vi "labviewArduino_1.vi"() -> ()   [LabVIEW 2017]
uses:
  <vilib>/MakerHub/LINX/Public/Peripherals/Digital/Digital Write N Chans.vi
  <vilib>/MakerHub/LINX/Private/Local IO/LinxDigitalWrite.vi
  <vilib>/MakerHub/LINX/Public/Utilities/Check Channel.vi
  <vilib>/MakerHub/LINX/Public/Utilities/Open Serial.vi
  <vilib>/MakerHub/LINX/Private/Utilties/Generate Error.vi
  <vilib>/Utility/file.llb/Write To Spreadsheet File (DBL).vi
  <vilib>/MakerHub/LINX/LMH-LINX.lvlib
panel:
  out "error out":errorcluster
  out "Result (V - I)":dbl[][](array[numeric]) format="%^#.6e"
  out "XY Graph 3":cluster{dbl[], dbl[]}(graph)
  in  "SweepSettings":T1 {"Vstep (V)" format="%.3f"; "Vstop (V)" format="%.3f"; "Vstart (V)" format="%.3f"}
  in  "Amount of modules connected":enum16{"1", "2", "3", "4", "5", "6"}(ring)
  in  "Start Button":bool
  in  "Time between measurements(s)":u32
  in  "Stop Button 2":bool
  in  "Time High Voltage Source is active (s)":u32
  in  "High voltage Source polarity":enum16{"-0+", "0-+", "-+0", "+0-"}(ring)
  out "Loop Rate (Hz)":u32
  in  "Serial Port":refnum<visa-resource-name>
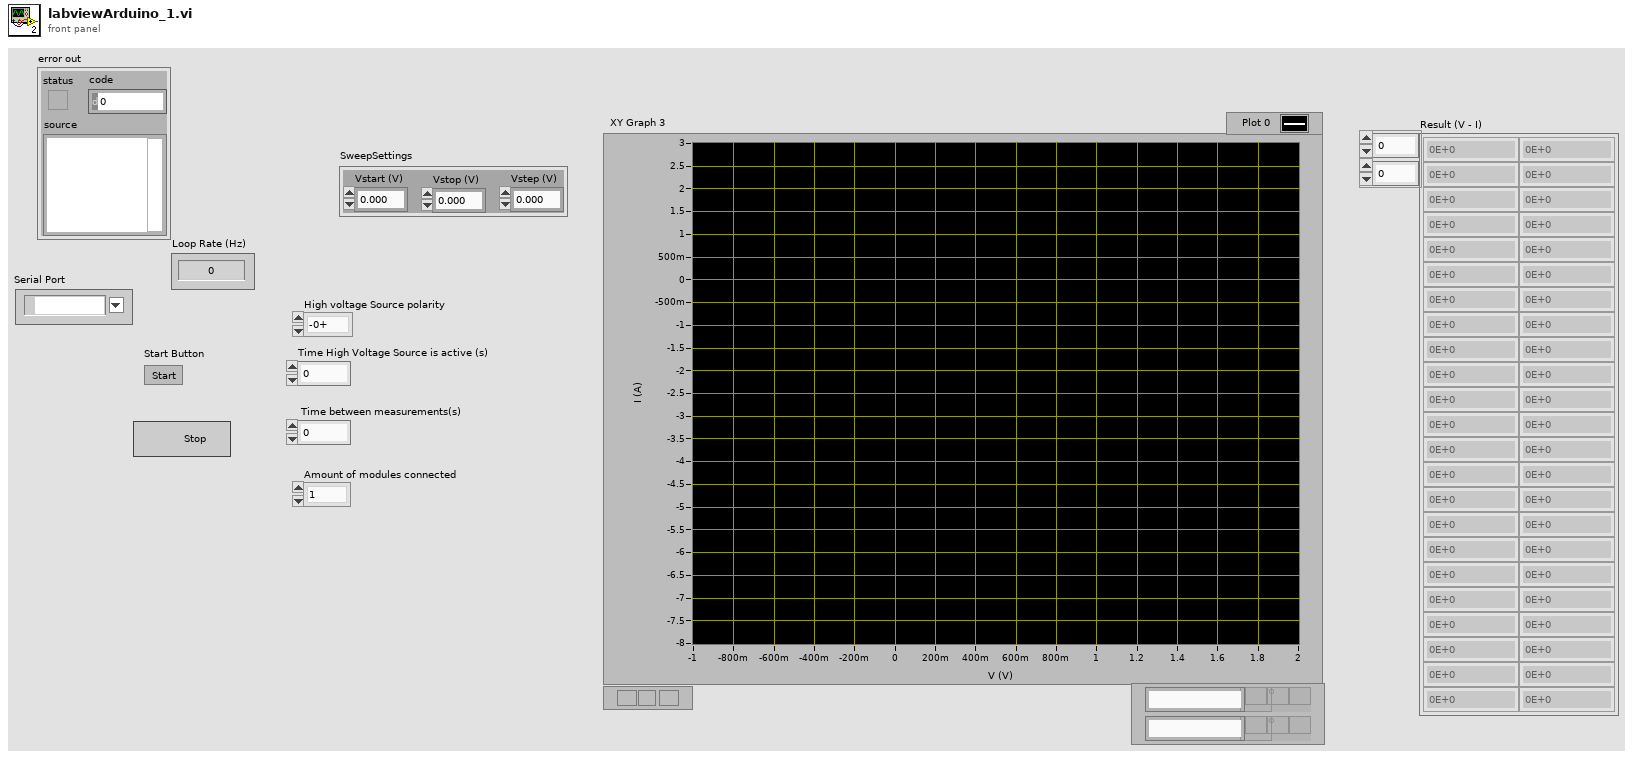
[diagram p1: front panel]
types:
  T1 = cluster{"Vstart (V)":dbl, "Vstop (V)":dbl, "Vstep (V)":dbl}
  T2 = enum16{"Rest", "HV Source On", "Measure", "Relay 1", "Relay 2", "Relay 3", "Relay 4", "Relay 5", "Relay 6"}
  T3 = enum16{"Rest", "HV Source On", "Relay 1", "Relay 2", "Relay 3", "Relay 4", "Relay 5", "Relay 6"}
  T4 = typedef "LMH-LINX.lvlib/LINX Ref.ctl" = cluster{"IO":T5, "Interface":T6, "LINX Device Config":T7}
  T5 = typedef "LMH-LINX.lvlib/Platform.ctl" = enum16{"Remote", "Local"}
  T6 = typedef "LMH-LINX.lvlib/Interface.ctl" = enum16{"Serial", "TCP"}
  T7 = typedef "LMH-LINX.lvlib/Device.lvlib/LINX Device Config.ctl" = cluster{"Interface":T6, "COM Port":refnum<visa-resource-name>, "TCP Configuration":T8, "Device Family":u8, "Device ID":u8, "Device Name":string, "TCP Ref":refnum<k5>, "Channels":T9}
  T8 = typedef "LMH-LINX.lvlib/Device.lvlib/TCP Config.ctl" = cluster{"IP Address":string, "Port":u16}
  T9 = typedef "LMH-LINX.lvlib/Channels.ctl" = cluster{"DI":u8[], "DO":u8[], "AI":u8[], "AO":u8[], "PWM":u8[], "QE":u8[], "UART":u8[], "I2C 2":u8[], "SPI":u8[], "CAN":u8[], "Servo":u8[], "AI Ref (V)":dbl, "AI Resolution (Bits)":u8, "AO Ref (V)":dbl, "AO Resolution (Bits)":u8}
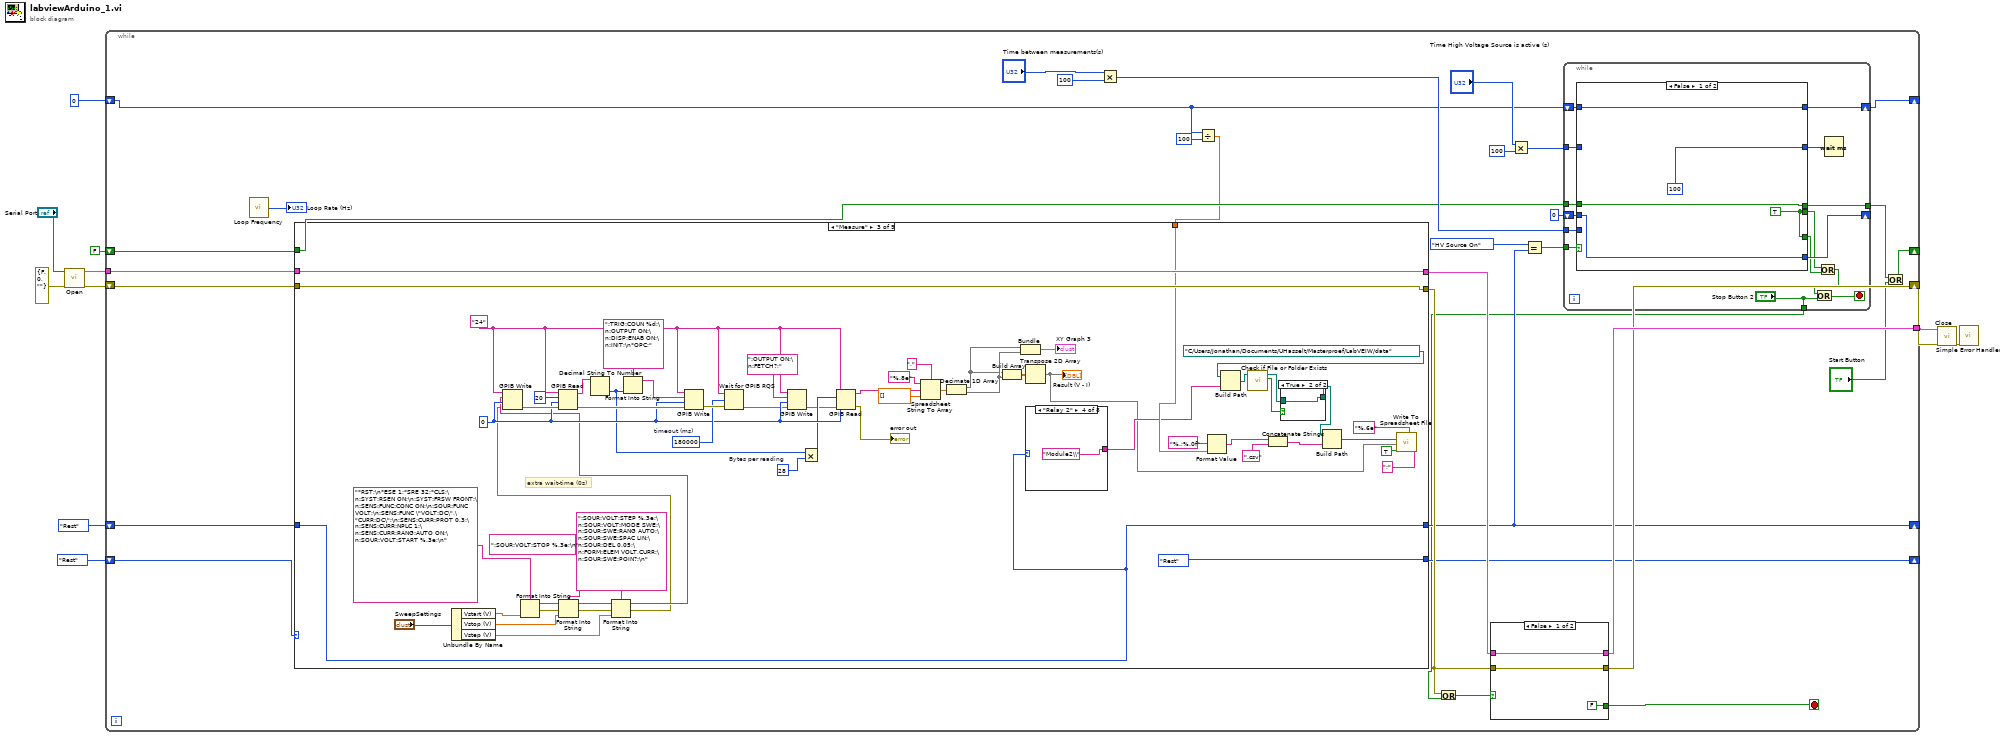
[diagram p0: block diagram]
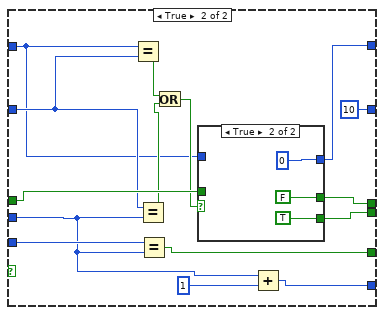
[diagram p2: hidden frame]
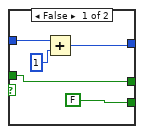
[diagram p3: hidden frame]
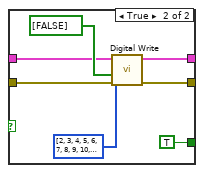
[diagram p4: hidden frame]
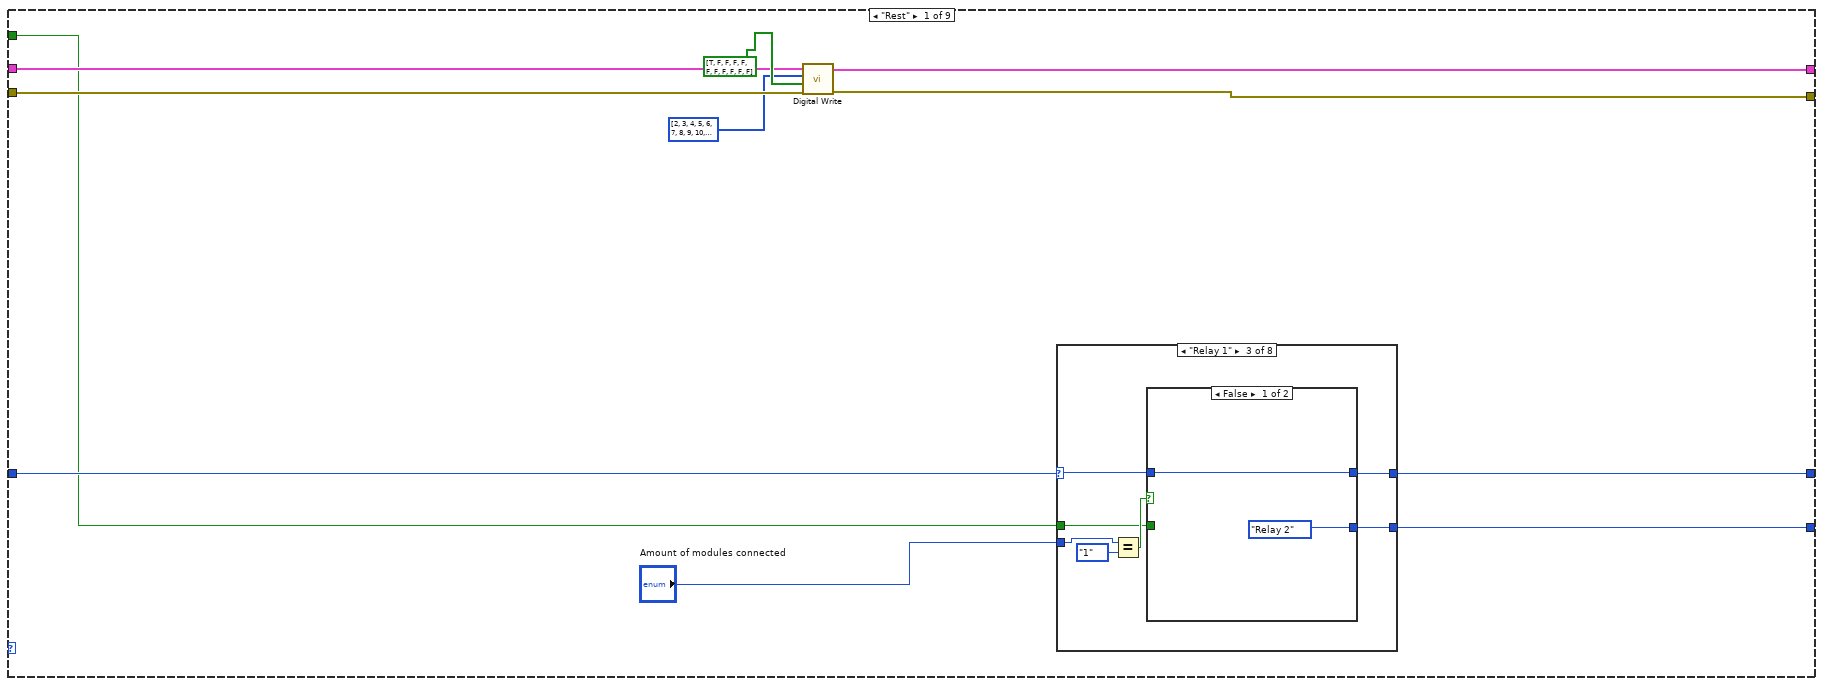
[diagram p5: hidden frame]
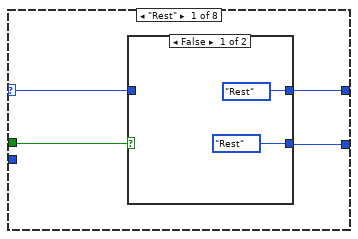
[diagram p6: hidden frame]
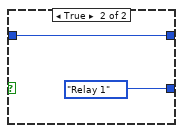
[diagram p7: hidden frame]
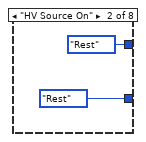
[diagram p8: hidden frame]
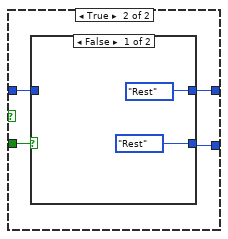
[diagram p9: hidden frame]
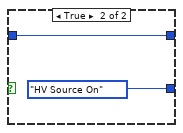
[diagram p10: hidden frame]
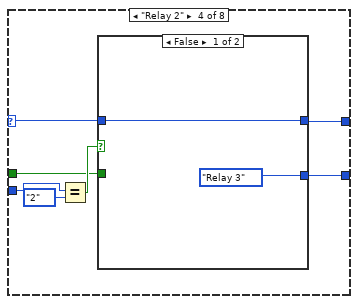
[diagram p11: hidden frame]
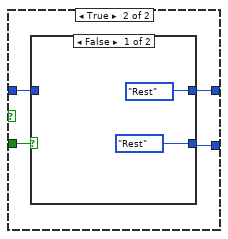
[diagram p12: hidden frame]
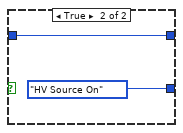
[diagram p13: hidden frame]
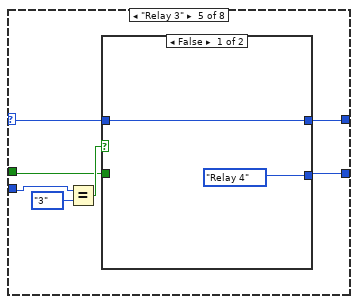
[diagram p14: hidden frame]
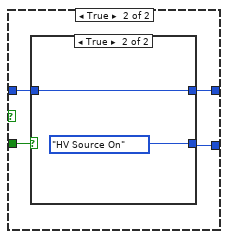
[diagram p15: hidden frame]
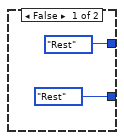
[diagram p16: hidden frame]
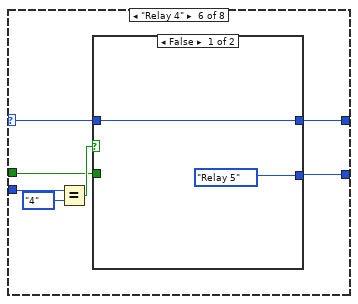
[diagram p17: hidden frame]
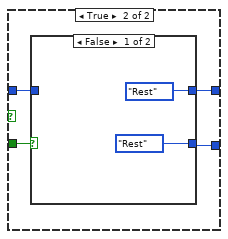
[diagram p18: hidden frame]
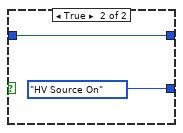
[diagram p19: hidden frame]
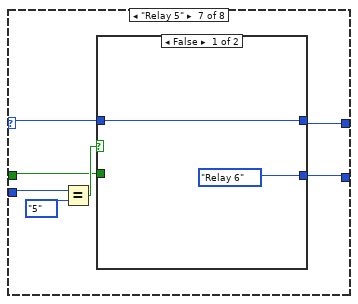
[diagram p20: hidden frame]
diagram:
  n1 = call-poly <vilib>:"Open.vi"("Error In"=errorcluster {"status"=FALSE, "code"=0, "source"=""}, "Serial Port"="Serial Port") -> ("Error Out"=w10:errorcluster, "LINX Resource"=w11:T4)  [unwired: 7 in, 1 out]
  n2 = while {
    tunnel: w11 -> [w41]
    tunnel: [w36] -> w9
    shift-right: [w35] -> w8
    shift-left: w10 -> [w40]
    shift-right: [w32] -> _
    shift-left: T2."Rest" ("Enum 2") -> [w17]
    shift-right: [w31] -> _
    shift-left: T3."Rest" ("Enum 2") -> [w33]
    shift-right: [w18] -> _
    shift-left: u32 0 ("y") -> [w14]
    shift-right: [w16] -> _
    shift-left: FALSE -> [w15]
    stop <- w27 stop-if-true
    n3 = call <vilib>:"Loop Frequency.vi"() -> ("Loop Rate (Hz)"=→"Loop Rate (Hz)":u32)
    n4 = Multiply(x="Time between measurements(s)", y=u32 100) -> (x*y=w21:u32)
    n5 = Divide(x=w14, y=u32 100) -> (x/y=w12:dbl)
    n6 = case shown="\"Measure\"" w17 {
      tunnel: [w106 T2."Rest" ("Enum 2") T2."Rest" ("Enum 2") T2."Measure" ("Enum 2") T2."Measure" ("Enum 2") T2."Measure" ("Enum 2") T2."Measure" ("Enum 2") T2."Measure" ("Enum 2") T2."Measure" ("Enum 2")] -> w32
      tunnel: w41 -> [w104 w231 w313 w331 w337 w347 w355 w363 w371]
      tunnel: w40 -> [w103 w230 w312 w330 w336 w346 w354 w362 w370]
      tunnel: [w102 w229 w312 w329 w338 w345 w352 w361 w369] -> w37
      tunnel: [w101 w226 w313 w328 w339 w344 w353 w360 w368] -> w38
      tunnel: [w99 T3."HV Source On" ("Enum 2") w311 T3."Relay 1" ("Enum 2") T3."Relay 2" ("Enum 2") T3."Relay 3" ("Enum 2") T3."Relay 4" ("Enum 2") T3."Relay 5" ("Enum 2") T3."Relay 6" ("Enum 2")] -> w31
      tunnel: w33 -> [w100 _ w311 _ _ _ _ _ _]
      tunnel: w15 -> [w98 _ _ _ _ _ _ _ _]
      tunnel: w12 -> [_ _ w306 _ _ _ _ _ _]
      frame "Rest" {
        n7 = call-poly <vilib>:"Digital Write.vi"("Error In"=w103, "Values"=bool[] [TRUE, FALSE, FALSE, FALSE, FALSE, FALSE, FALSE, FALSE, FALSE, FALSE, FALSE], "DO Channels"=u8[] [2, 3, 4, 5, 6, 7, 8, 9, 10, 11, 12, 13], "LINX Resource"=w104) -> ("Error Out"=w102:errorcluster, "LINX Resource"=w101:T4)  [unwired: 6 in]
        n8 = case shown="\"Relay 1\"" w100 {
          selector: w100 -> [w109 _ w119 w138 w155 w169 w187 w207]
          tunnel: [w108 T2."Rest" ("Enum 2") w118 w135 w152 w171 w189 w208] -> w106
          tunnel: [w110 T3."Rest" ("Enum 2") w117 w136 w153 w172 w188 w206] -> w99
          tunnel: w98 -> [w107 _ w120 w137 w154 w170 w186 w205]
          tunnel: "Amount of modules connected" -> [_ _ w121 w134 w151 w168 w185 w204]
          frame "Rest" {
            n9 = case shown="False" w107 {
              tunnel: [T2."Rest" ("Enum 2") T2."Relay 1" ("Enum 2")] -> w108
              tunnel: [T3."Rest" ("Enum 2") w113] -> w110
              tunnel: w109 -> [_ w113]
              frame False {
              }
              frame True {
              }
            }
          }
          frame "HV Source On" {
          }
          frame "Relay 1" {
            n10 = Equal?(x=w121, y=enum16{"1", "2", "3", "4", "5", "6"}."1") -> (x = y?=w122:bool)
            n11 = case shown="False" w122 {
              tunnel: [T2."Relay 2" ("Enum 2") w129] -> w118
              tunnel: w119 -> [w125 w128]
              tunnel: [w125 w127] -> w117
              tunnel: w120 -> [_ w126]
              frame False {
              }
              frame True {
                n12 = case shown="False" w126 {
                  tunnel: [T2."Rest" ("Enum 2") T2."HV Source On" ("Enum 2")] -> w129
                  tunnel: [T3."Rest" ("Enum 2") w133] -> w127
                  tunnel: w128 -> [_ w133]
                  frame False {
                  }
                  frame True {
                  }
                }
              }
            }
          }
          frame "Relay 2" {
            n13 = Equal?(x=w134, y=enum16{"1", "2", "3", "4", "5", "6"}."2") -> (x = y?=w139:bool)
            n14 = case shown="False" w139 {
              tunnel: [T2."Relay 3" ("Enum 2") w146] -> w135
              tunnel: w138 -> [w142 w145]
              tunnel: [w142 w144] -> w136
              tunnel: w137 -> [_ w143]
              frame False {
              }
              frame True {
                n15 = case shown="False" w143 {
                  tunnel: [T2."Rest" ("Enum 2") T2."HV Source On" ("Enum 2")] -> w146
                  tunnel: [T3."Rest" ("Enum 2") w150] -> w144
                  tunnel: w145 -> [_ w150]
                  frame False {
                  }
                  frame True {
                  }
                }
              }
            }
          }
          frame "Relay 3" {
            n16 = Equal?(x=w151, y=enum16{"1", "2", "3", "4", "5", "6"}."3") -> (x = y?=w156:bool)
            n17 = case shown="False" w156 {
              tunnel: [T2."Relay 4" ("Enum 2") w163] -> w152
              tunnel: w155 -> [w159 w162]
              tunnel: [w159 w161] -> w153
              tunnel: w154 -> [_ w160]
              frame False {
              }
              frame True {
                n18 = case shown="True" w160 {
                  tunnel: [T2."Rest" ("Enum 2") T2."HV Source On" ("Enum 2")] -> w163
                  tunnel: [T3."Rest" ("Enum 2") w167] -> w161
                  tunnel: w162 -> [_ w167]
                  frame False {
                  }
                  frame True {
                  }
                }
              }
            }
          }
          frame "Relay 4" {
            n19 = Equal?(x=w168, y=enum16{"1", "2", "3", "4", "5", "6"}."4") -> (x = y?=w173:bool)
            n20 = case shown="False" w173 {
              tunnel: [T2."Relay 5" ("Enum 2") w180] -> w171
              tunnel: w169 -> [w176 w179]
              tunnel: [w176 w178] -> w172
              tunnel: w170 -> [_ w177]
              frame False {
              }
              frame True {
                n21 = case shown="False" w177 {
                  tunnel: [T2."Rest" ("Enum 2") T2."HV Source On" ("Enum 2")] -> w180
                  tunnel: [T3."Rest" ("Enum 2") w184] -> w178
                  tunnel: w179 -> [_ w184]
                  frame False {
                  }
                  frame True {
                  }
                }
              }
            }
          }
          frame "Relay 5" {
            n22 = Equal?(x=w185, y=enum16{"1", "2", "3", "4", "5", "6"}."5") -> (x = y?=w190:bool)
            n23 = case shown="False" w190 {
              tunnel: [T2."Relay 6" ("Enum 2") w197] -> w189
              tunnel: w187 -> [w193 w196]
              tunnel: [w193 w195] -> w188
              tunnel: w186 -> [_ w194]
              frame False {
              }
              frame True {
                n24 = case shown="False" w194 {
                  tunnel: [T2."Rest" ("Enum 2") T2."HV Source On" ("Enum 2")] -> w197
                  tunnel: [T3."Rest" ("Enum 2") w201] -> w195
                  tunnel: w196 -> [_ w201]
                  frame False {
                  }
                  frame True {
                  }
                }
              }
            }
          }
          frame "Relay 6" {
            n25 = Equal?(x=w204, y=enum16{"1", "2", "3", "4", "5", "6"}."6") -> (x = y?=w202:bool)
            n26 = case shown="False" w202 {
              tunnel: [w210 w220] -> w208
              tunnel: w207 -> [w212 w219]
              tunnel: [w209 w218] -> w206
              tunnel: w205 -> [w211 w217]
              frame False {
                n27 = case shown="False" w211 {
                  tunnel: [T2."Rest" ("Enum 2") T2."HV Source On" ("Enum 2")] -> w210
                  tunnel: [T3."Rest" ("Enum 2") w216] -> w209
                  tunnel: w212 -> [_ w216]
                  frame False {
                  }
                  frame True {
                  }
                }
              }
              frame True {
                n28 = case shown="False" w217 {
                  tunnel: [T2."Rest" ("Enum 2") T2."HV Source On" ("Enum 2")] -> w220
                  tunnel: [T3."Rest" ("Enum 2") w224] -> w218
                  tunnel: w219 -> [_ w224]
                  frame False {
                  }
                  frame True {
                  }
                }
              }
            }
          }
        }
      }
      frame "HV Source On" {
        n29 = case shown="\"-0+\", Default" "High voltage Source polarity" {
          tunnel: w231 -> [w234 w241 w247 w253]
          tunnel: w230 -> [w235 w240 w244 w252]
          tunnel: [w233 w239 w246 w250] -> w226
          tunnel: [w232 w238 w245 w251] -> w229
          frame "-0+", Default {
            n30 = call-poly <vilib>:"Digital Write.vi"("Error In"=w235, "Values"=bool[] [FALSE, FALSE, FALSE, FALSE, FALSE, FALSE, FALSE, FALSE, TRUE, TRUE, TRUE], "DO Channels"=u8[] [2, 3, 4, 5, 6, 7, 8, 9, 10, 11, 12, 13], "LINX Resource"=w234) -> ("Error Out"=w232:errorcluster, "LINX Resource"=w233:T4)  [unwired: 6 in]
          }
          frame "0-+" {
            n31 = call-poly <vilib>:"Digital Write.vi"("Error In"=w240, "Values"=bool[] [FALSE, FALSE, FALSE, FALSE, FALSE, FALSE, FALSE, FALSE, FALSE, TRUE, TRUE, TRUE], "DO Channels"=u8[] [2, 3, 4, 5, 6, 7, 8, 9, 10, 11, 12, 13], "LINX Resource"=w241) -> ("Error Out"=w238:errorcluster, "LINX Resource"=w239:T4)  [unwired: 6 in]
          }
          frame "-+0" {
            n32 = call-poly <vilib>:"Digital Write.vi"("Error In"=w244, "Values"=bool[] [FALSE, FALSE, FALSE, FALSE, FALSE, FALSE, FALSE, FALSE, TRUE, TRUE, FALSE, TRUE], "DO Channels"=u8[] [2, 3, 4, 5, 6, 7, 8, 9, 10, 11, 12, 13], "LINX Resource"=w247) -> ("Error Out"=w245:errorcluster, "LINX Resource"=w246:T4)  [unwired: 6 in]
          }
          frame "+0-" {
            n33 = call-poly <vilib>:"Digital Write.vi"("Error In"=w252, "Values"=bool[] [FALSE, FALSE, FALSE, FALSE, FALSE, FALSE, FALSE, FALSE, TRUE, FALSE, TRUE, TRUE], "DO Channels"=u8[] [2, 3, 4, 5, 6, 7, 8, 9, 10, 11, 12, 13], "LINX Resource"=w253) -> ("Error Out"=w251:errorcluster, "LINX Resource"=w250:T4)  [unwired: 6 in]
          }
        }
      }
      frame "Measure" {
        w284 = "24" ("address string")
        w288 = 28  # Bytes per reading
        w292 = 180000  # timeout (ms)
        w290 = i16 0 ("mode (0)")
        # "extra wait-time (0s)"
        n34 = Unbundle By Name("SweepSettings") -> ("Vstart (V)"=w273:dbl, "Vstop (V)"=w272:dbl, "Vstep (V)"=w274:dbl)
        n35 = Format Into String(format string="*RST;\n*ESE 1;*SRE 32;*CLS;\n:SYST:RSEN ON;\n:SYST:FRSW FRONT;\n:SENS:FUNC:CONC ON;\n:SOUR:FUNC VOLT;\n:SENS:FUNC \"VOLT:DC\",\"CURR:DC\";\n:SENS:CURR:PROT 0.3;\n:SENS:CURR:NPLC 1;\n:SENS:CURR:RANG:AUTO ON;\n:SOUR:VOLT:START %.3e;\n", w273) -> (resulting string=w268:string, error out=w269:errorcluster)  [unwired: 2 in]
        n36 = Format Into String(format string=":SOUR:VOLT:STOP %.3e;\n", initial string=w268, error in=w269, w272) -> (resulting string=w270:string, error out=w271:errorcluster)
        n37 = Format Into String(format string=":SOUR:VOLT:STEP %.3e;\n:SOUR:VOLT:MODE SWE;\n:SOUR:SWE:RANG AUTO;\n:SOUR:SWE:SPAC LIN;\n:SOUR:DEL 0.05;\n:FORM:ELEM VOLT,CURR;\n:SOUR:SWE:POIN?;\n", initial string=w270, error in=w271, w274) -> (resulting string=w263:string, error out=w262:errorcluster)
        n38 = GPIB Write(0:w284, 1:w263, 2:w290, 3:w262) -> (6:w298:errorcluster)  [unwired: 1 in, 1 out]
        n39 = GPIB Read(0:w284, 1:20 ("byte count"), 2:w290, 3:w298) -> (5:w295:string, 7:w294:errorcluster)  [unwired: 1 in, 1 out]
        n40 = Decimal String To Number(string=w295) -> (number=w289:i32)  [unwired: 2 in, 1 out]
        n41 = Format Into String(format string=":TRIG:COUN %d;\n:OUTPUT ON;\n:DISP:ENAB ON;\n:INIT;\n*OPC;", w289) -> (resulting string=w296:string)  [unwired: 2 in, 1 out]
        n42 = GPIB Write(0:w284, 1:w296, 2:w290, 3:w294) -> (6:w293:errorcluster)  [unwired: 1 in, 1 out]
        n43 = Wait for GPIB RQS(2:w293, 3:w292, 4:w284) -> (0:w286:errorcluster)  [unwired: 1 out]
        n44 = GPIB Write(0:w284, 1:":OUTPUT ON;\n:FETCH?;", 2:w290, 3:w286) -> (6:w285:errorcluster)  [unwired: 1 in, 1 out]
        n45 = Multiply(x=w289, y=w288) -> (x*y=w287:i32)
        n46 = GPIB Read(0:w284, 1:w287, 2:w290, 3:w285) -> (5:w279:string, 7:→"error out":errorcluster)  [unwired: 1 in, 1 out]
        n47 = Spreadsheet String To Array(delimiter (Tab)=",", format string="%.8e", spreadsheet string=w279, array type (2D Dbl)=dbl[] []) -> (array=w280:dbl[])
        n48 = Decimate 1D Array(w280) -> (w276:dbl[], w277:dbl[])
        n49 = Build Array(w276, w277) -> (w278:dbl[][])
        n50 = Bundle(w276, w277) -> (→"XY Graph 3":cluster{dbl[], dbl[]})  [unwired: 1 in]
        n51 = case shown="\"Relay 2\"" w311 {
          tunnel: ["fault" ("name or relative path") "fault" ("name or relative path") "Module1" ("name or relative path") "Module2\\" ("name or relative path") "Module3\\" ("name or relative path") "Module4\\" ("name or relative path") "Module5\\" ("name or relative path") "Module6\\" ("name or relative path")] -> w304
          frame "Rest" {
          }
          frame "HV Source On" {
          }
          frame "Relay 1" {
          }
          frame "Relay 2" {
          }
          frame "Relay 3" {
          }
          frame "Relay 4" {
          }
          frame "Relay 5" {
          }
          frame "Relay 6" {
          }
        }
        n52 = Transpose 2D Array(2D array=w278) -> (transposed array=w259:dbl[][])
        "Result (V - I)" <- w259
        n53 = Format Value(format string="%.;%.0f", value (0)=w306) -> (output string=w310:string)  [unwired: 1 in]
        n54 = Build Path(base path=path "C:/Users/Jonathan/Documents/UHasselt/Masterproef/LabVEIW/data", name or relative path=w304) -> (appended path=w303:path)
        n55 = call <vilib>:"Check if File or Folder Exists.vi"("path"=w303) -> ("file or folder exists?"=w302:bool, "dup path"=w301:path)  [unwired: 8 in, 1 out]
        n56 = Concatenate Strings(w310, ".csv" ("string")) -> (w309:string)
        n57 = case shown="True" w302 {
          tunnel: w301 -> [w316 w317]
          tunnel: [w315 w317] -> w300
          frame False {
            n58 = Create Folder(path (use dialog)=w316) -> (created path=w315:path)  [unwired: 2 in, 2 out]
          }
          frame True {
          }
        }
        n59 = Build Path(base path=w300, name or relative path=w309) -> (appended path=w260:path)
        n60 = call-poly <vilib>:"Write To Spreadsheet File.vi"("delimiter (\\t)"=";" ("delimiter (\\t)"), "format (%.3f)"="%.6e", "append to file? (new file:F)"=TRUE, "2D data"=w259, "file path (dialog if empty)"=w260) -> ()  [unwired: 3 in, 1 out]
      }
      frame "Relay 1" {
        n61 = call-poly <vilib>:"Digital Write.vi"("Error In"=w330, "Values"=bool[] [FALSE, TRUE, FALSE, FALSE, FALSE, FALSE, FALSE, TRUE, FALSE, FALSE, FALSE], "DO Channels"=u8[] [2, 3, 4, 5, 6, 7, 8, 9, 10, 11, 12, 13], "LINX Resource"=w331) -> ("Error Out"=w329:errorcluster, "LINX Resource"=w328:T4)  [unwired: 6 in]
      }
      frame "Relay 2" {
        n62 = call-poly <vilib>:"Digital Write.vi"("Error In"=w336, "Values"=bool[] [FALSE, FALSE, TRUE, FALSE, FALSE, FALSE, FALSE, TRUE, FALSE, FALSE, FALSE], "DO Channels"=u8[] [2, 3, 4, 5, 6, 7, 8, 9, 10, 11, 12, 13], "LINX Resource"=w337) -> ("Error Out"=w338:errorcluster, "LINX Resource"=w339:T4)  [unwired: 6 in]
      }
      frame "Relay 3" {
        n63 = call-poly <vilib>:"Digital Write.vi"("Error In"=w346, "Values"=bool[] [FALSE, FALSE, FALSE, TRUE, FALSE, FALSE, FALSE, TRUE, FALSE, FALSE, FALSE], "DO Channels"=u8[] [2, 3, 4, 5, 6, 7, 8, 9, 10, 11, 12, 13], "LINX Resource"=w347) -> ("Error Out"=w345:errorcluster, "LINX Resource"=w344:T4)  [unwired: 6 in]
      }
      frame "Relay 4" {
        n64 = call-poly <vilib>:"Digital Write.vi"("Error In"=w354, "Values"=bool[] [FALSE, FALSE, FALSE, FALSE, TRUE, FALSE, FALSE, TRUE, FALSE, FALSE, FALSE], "DO Channels"=u8[] [2, 3, 4, 5, 6, 7, 8, 9, 10, 11, 12, 13], "LINX Resource"=w355) -> ("Error Out"=w352:errorcluster, "LINX Resource"=w353:T4)  [unwired: 6 in]
      }
      frame "Relay 5" {
        n65 = call-poly <vilib>:"Digital Write.vi"("Error In"=w362, "Values"=bool[] [FALSE, FALSE, FALSE, FALSE, FALSE, TRUE, FALSE, TRUE, FALSE, FALSE, FALSE], "DO Channels"=u8[] [2, 3, 4, 5, 6, 7, 8, 9, 10, 11, 12, 13], "LINX Resource"=w363) -> ("Error Out"=w361:errorcluster, "LINX Resource"=w360:T4)  [unwired: 6 in]
      }
      frame "Relay 6" {
        n66 = call-poly <vilib>:"Digital Write.vi"("Error In"=w370, "Values"=bool[] [FALSE, FALSE, FALSE, FALSE, FALSE, FALSE, TRUE, TRUE, FALSE, FALSE, FALSE], "DO Channels"=u8[] [2, 3, 4, 5, 6, 7, 8, 9, 10, 11, 12, 13], "LINX Resource"=w371) -> ("Error Out"=w369:errorcluster, "LINX Resource"=w368:T4)  [unwired: 6 in]
      }
    }
    n67 = Multiply(x="Time High Voltage Source is active (s)", y=u32 100) -> (x*y=w24:u32)
    n68 = Equal?(x=T3."HV Source On", y=w31) -> (x = y?=w30:bool)
    n69 = while {
      tunnel: w30 -> [w57]
      tunnel: w24 -> [w56]
      shift-right: [w54] -> _
      shift-left: u32 0 ("y") -> [w53]
      tunnel: ["Stop Button 2"] -> w28
      tunnel: w21 -> [w50]
      tunnel: [w46] -> w20
      tunnel: w15 -> [w45]
      shift-right: [w43] -> w18
      shift-left: w14 -> [w44]
      stop <- w52 stop-if-true
      n70 = case shown="False" w57 {
        tunnel: [u32 100 ("millisecond multiple") u32 10 ("millisecond multiple")] -> w55
        tunnel: w56 -> [_ w68]
        tunnel: w53 -> [w61 w73]
        tunnel: [w60 w71] -> w49
        tunnel: [w61 w75] -> w54
        tunnel: w50 -> [_ w74]
        tunnel: [w60 w72] -> w48
        tunnel: [w59 w70] -> w46
        tunnel: w45 -> [w59 w69]
        tunnel: w44 -> [w58 w63]
        tunnel: [w58 w64] -> w43
        frame False {
          w60 = TRUE
        }
        frame True {
          n71 = Equal?(x=w63, y=w68) -> (x = y?=w67:bool)
          n72 = Equal?(x=w68, y=w73) -> (x = y?=w65:bool)
          n73 = Equal?(x=w74, y=w73) -> (x = y?=w72:bool)
          n74 = Or(x=w67, y=w65) -> (x .or. y?=w66:bool)
          n75 = case shown="True" w66 {
            tunnel: [FALSE TRUE] -> w71
            tunnel: [w81 FALSE] -> w70
            tunnel: w69 -> [w81 _]
            tunnel: [w80 0] -> w64
            tunnel: w63 -> [w79 _]
            frame False {
              n76 = Add(x=w79, y=u32 1 ("millisecond multiple")) -> (x+y=w80:u32)
            }
            frame True {
            }
          }
          n77 = Add(x=w73, y=1) -> (x+y=w75:u32)
        }
      }
      n78 = Or(x=w49, y=w48) -> (x .or. y?=w47:bool)
      n79 = Or(x=w47, y="Stop Button 2") -> (x .or. y?=w52:bool)
      n80 = Wait (ms)(milliseconds to wait=w55) -> ()  [unwired: 1 out]
    }
    n81 = Or(x=w37, y=w28) -> (x .or. y?=w39:bool)
    n82 = case shown="False" w39 {
      tunnel: w38 -> [w88 w93]
      tunnel: [w88 w92] -> w36
      tunnel: [w87 w91] -> w35
      tunnel: w37 -> [w87 w90]
      tunnel: [FALSE TRUE] -> w27
      frame False {
      }
      frame True {
        n83 = call-poly <vilib>:"Digital Write.vi"("Error In"=w90, "Values"=bool[] [FALSE], "DO Channels"=u8[] [2, 3, 4, 5, 6, 7, 8, 9, 10, 11, 12, 13], "LINX Resource"=w93) -> ("Error Out"=w91:errorcluster, "LINX Resource"=w92:T4)  [unwired: 6 in]
      }
    }
    n84 = Or(x=w20, y="Start Button") -> (x .or. y?=w16:bool)
  }
  n85 = call <vilib>:"Close.vi"("Error In"=w8, "LINX Resource"=w9) -> ("Error Out"=w6:errorcluster)  [unwired: 9 in]
  n86 = call <vilib>:"Simple Error Handler.vi"("error in (no error)"=w6) -> ()  [unwired: 4 in, 5 out]
